vi "script_get_next_command.vi"(2 "Current index to read":i32, 3 "Script lines":string[](array[string])) -> (0 "Next index to read":i32, 1 "Command":string)   [LabVIEW 2010]
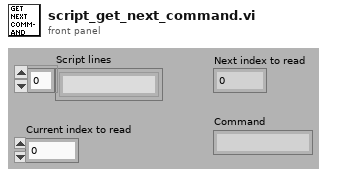
[diagram p1: front panel]
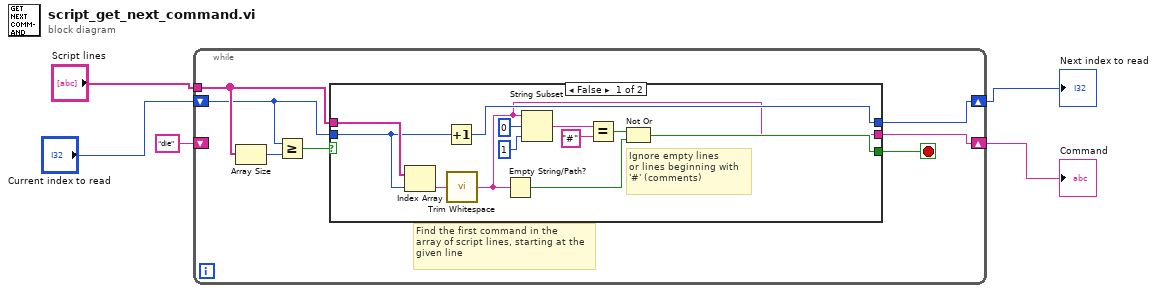
[diagram p0: block diagram]
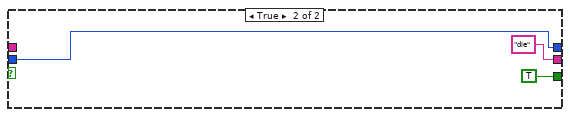
[diagram p2: hidden frame]
diagram:
  n1 = while {
    tunnel: "Script lines" -> [w9]
    shift-right: [w8] -> w3
    shift-left: "die" -> [_]
    shift-right: [w6] -> w5
    shift-left: "Current index to read" -> [w7]
    stop <- w10 stop-if-true
    # "Find the first command in the\narray of script lines, starting at the\ngiven line"
    n2 = Array Size(array=w9) -> (size(s)=w12:i32)
    n3 = Greater Or Equal?(x=w7, y=w12) -> (x >= y?=w11:bool)
    n4 = case shown="False" w11 {
      tunnel: [w13 "die"] -> w8
      tunnel: [w14 TRUE] -> w10
      tunnel: w9 -> [w24 _]
      tunnel: w7 -> [w16 w25]
      tunnel: [w15 w25] -> w6
      frame False {
        # "Ignore empty lines\nor lines beginning with\n'#' (comments)"
        n5 = Index Array(array=w24, index=w16) -> (element=w23:string)
        n6 = Increment(x=w16) -> (x+1=w15:i32)
        n7 = call <vilib>:"Trim Whitespace.vi"("string"=w23) -> ("trimmed string"=w13:string)  [unwired: 1 in]
        n8 = Empty String/Path?(string/path=w13) -> (empty?=w18:bool)
        n9 = String Subset(string=w13, offset (0)=0, length (rest)=1 ("length (rest)")) -> (substring=w17:string)
        n10 = Equal?(x=w17, y="#") -> (x = y?=w19:bool)
        n11 = Not Or(1:w18, 2:w19) -> (0:w14:bool)
      }
      frame True {
      }
    }
  }
  "Next index to read" <- w5
  "Command" <- w3
